vi "StartData.vi"(8 "error in (no error)":errorcluster, 11 "Class In":refnum<class "SensorBase.lvclass">) -> (0 "error out":errorcluster, 3 "Class Out":refnum<class "SensorBase.lvclass">)   [LabVIEW 2014, in "SensorPlugins.lvlib" / "SensorBase.lvclass"]
uses:
  SensorBase.lvclass
  <userlib>/NIST/BaseClasses/Object_class/BaseObject.lvclass
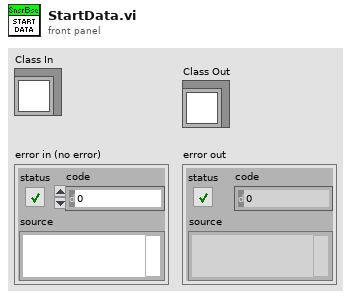
[diagram p1: front panel]
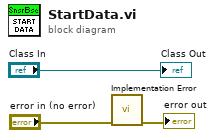
[diagram p0: block diagram]
diagram:
  n1 = call <userlib>:"Implementation Error.vi"("error in (no error)"="error in (no error)") -> ("error out"=→"error out":errorcluster)  [unwired: 10 in]
  "Class Out" <- "Class In"
